vi "CalculateInformation.vi"(8 "error in":errorcluster, 9 "ImageIn":T1(plugin-control), 10 "Number of Particles":i32, 11 "Particle Measurements":dbl[][](array[numeric]) format="%.2f") -> (0 "error out":errorcluster, 1 "LinePoints":cluster{"X":i32, "Y":i32}[](array[cluster]), 2 "OverlayImageOut":T1(plugin-control), 3 "ScaleAngleDegrees":dbl)   [LabVIEW 2017]
panel:
  out "RightParticle":dbl[](array[numeric])
  out "LeftParticle":dbl[](array[numeric])
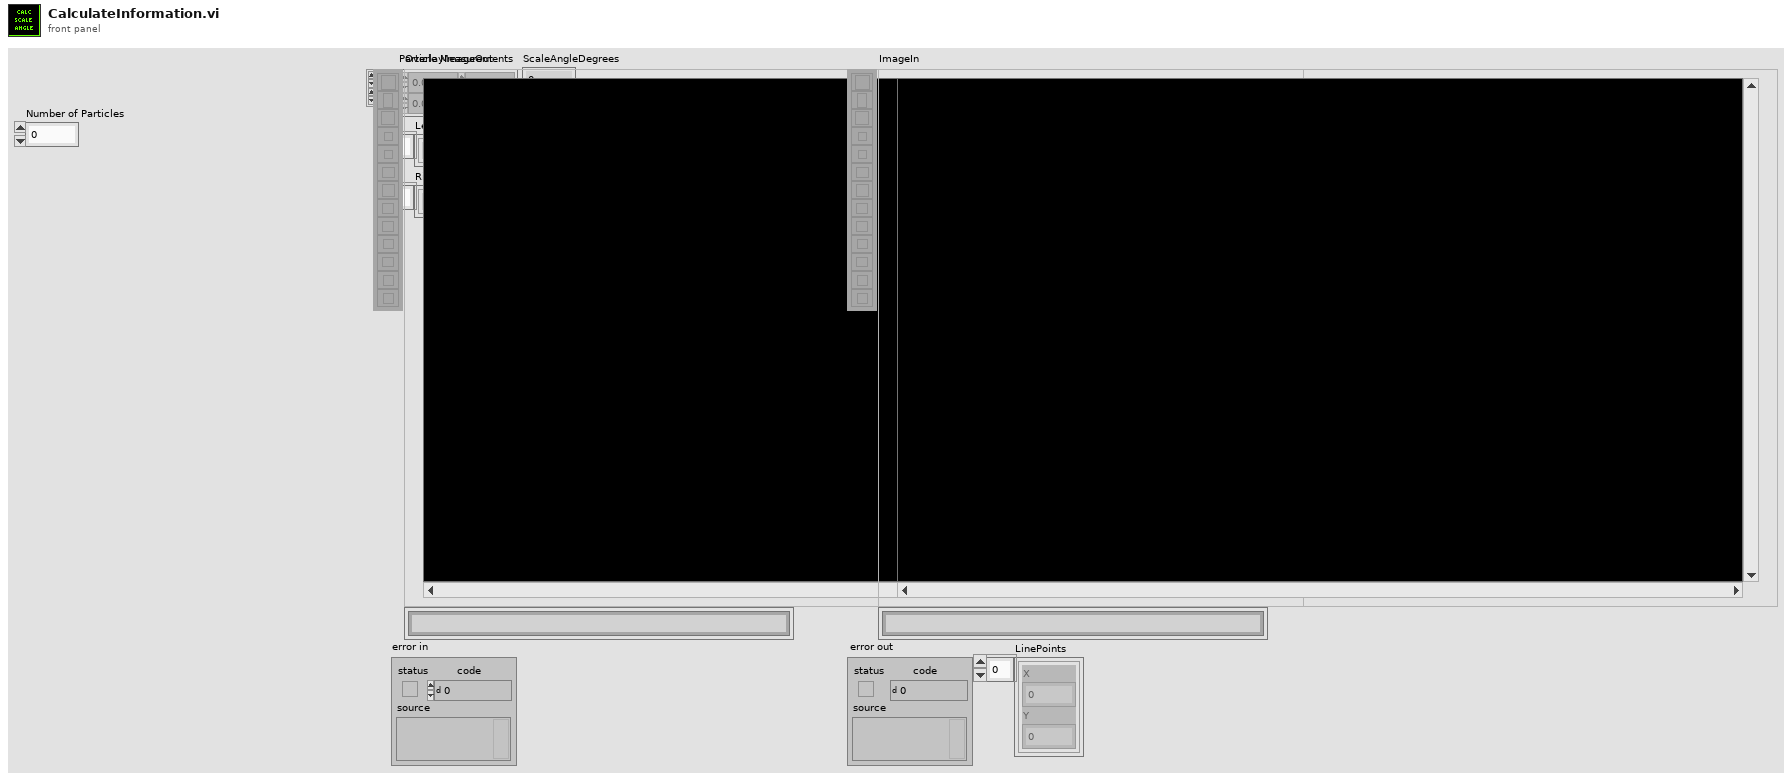
[diagram p1: front panel]
types:
  T1 = typedef "IMAQ Image.ctl" = refnum<image>
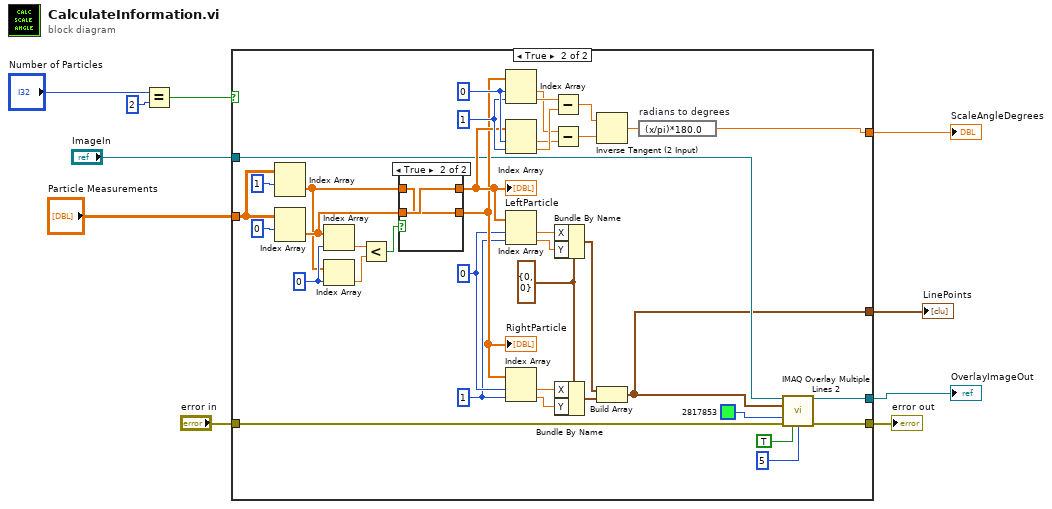
[diagram p0: block diagram]
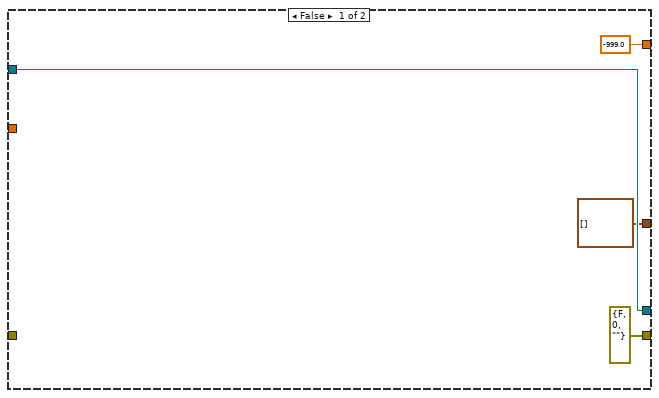
[diagram p2: hidden frame]
diagram:
  n1 = Equal?(x="Number of Particles", y=2) -> (x = y?=w8:bool)
  n2 = case shown="True" w8 {
    tunnel: "Particle Measurements" -> [_ w52]
    tunnel: [-999.0 w34] -> w6
    tunnel: "ImageIn" -> [w13 w22]
    tunnel: [w13 w18] -> w4
    tunnel: "error in" -> [_ w20]
    tunnel: [errorcluster {"status"=FALSE, "code"=0, "source"=""} ("error out") w19] -> w2
    tunnel: [cluster{"X":i32, "Y":i32}[] [] w15] -> w1
    frame False {
    }
    frame True {
      w28 = 1 ("index")
      w29 = 0 ("index")
      w25 = cluster{"X":i32, "Y":i32} {"X"=0, "Y"=0} ("Start Point")
      w42 = 1 ("index")
      w43 = 0 ("index")
      w49 = 0 ("index")
      n3 = Index Array(array=w52, index (row)=1) -> (element=w44:dbl[])  [unwired: 1 in]
      n4 = Index Array(array=w52, index (row)=0) -> (element=w45:dbl[])  [unwired: 1 in]
      n5 = Index Array(array=w45, index=w49) -> (element=w46:dbl)
      n6 = Index Array(array=w44, index=w49) -> (element=w48:dbl)
      n7 = Less?(x=w46, y=w48) -> (x < y?=w47:bool)
      n8 = case shown="True" w47 {
        tunnel: w45 -> [w54 w56]
        tunnel: [w53 w56] -> w33
        tunnel: w44 -> [w53 w55]
        tunnel: [w54 w55] -> w30
        frame False {
        }
        frame True {
        }
      }
      "LeftParticle" <- w33
      "RightParticle" <- w30
      n9 = Index Array(array=w30, index #1=w43, index #2=w42) -> (element #1=w38:dbl, element #2=w41:dbl)
      n10 = Index Array(array=w33, index #1=w43, index #2=w42) -> (element #1=w37:dbl, element #2=w40:dbl)
      n11 = Index Array(array=w33, index #1=w29, index #2=w28) -> (element #1=w32:dbl, element #2=w31:dbl)
      n12 = Index Array(array=w30, index #1=w29, index #2=w28) -> (element #1=w27:dbl, element #2=w26:dbl)
      n13 = Subtract(x=w41, y=w40) -> (x-y=w39:dbl)
      n14 = Subtract(x=w38, y=w37) -> (x-y=w36:dbl)
      n15 = Bundle By Name(cluster=w25, "X"=w32, "Y"=w31) -> (w24:cluster{"X":i32, "Y":i32})
      n16 = Bundle By Name(cluster=w25, "X"=w27, "Y"=w26) -> (w23:cluster{"X":i32, "Y":i32})
      n17 = Inverse Tangent (2 Input)(1:w36, 2:w39) -> (0:w35:dbl)
      n18 = Build Array(w24, w23) -> (w15:cluster{"X":i32, "Y":i32}[])
      n19 = expression code="(x/pi)*180.0" "radians to degrees"(w35) -> (w34:dbl)
      n20 = call "IMAQ Overlay Multiple Lines 2"("Image"=w22, "Line End Points"=w15, "Color"=u32 2817853, "error in (no error)"=w20, "Maintain Width?"=TRUE, "Width"=u32 5) -> ("Image Out"=w18:T1, "error out"=w19:errorcluster)  [unwired: 8 in]
    }
  }
  "ScaleAngleDegrees" <- w6
  "OverlayImageOut" <- w4
  "error out" <- w2
  "LinePoints" <- w1
